vi "get shared memory structs and definitions.vi"(7 "engine in":refnum<class "Engine Parent Editor Node.lvclass">, 8 "error in (no error)":errorcluster, 11 "editor node in":refnum<class "module editor node.lvclass">) -> (0 "error out":errorcluster, 1 "shm file definitions":string, 2 "shm data structs":string, 3 "editor node out":refnum<class "module editor node.lvclass">, 5 "engine out":refnum<class "Engine Parent Editor Node.lvclass">)   [LabVIEW 2014, in "Shared Memory editor node.lvclass"]
uses:
  Shared Memory editor node.lvclass
  <vilib>/NI/DCAF/Tag Editor Core/Configuration Editor/Classes/Engine Parent/Engine Parent Editor Node.lvclass
  <vilib>/NI/DCAF/Tag Editor Core/Configuration Editor/Classes/Module editor node/module editor node.lvclass
  cheddar/C Header Generator.lvlib
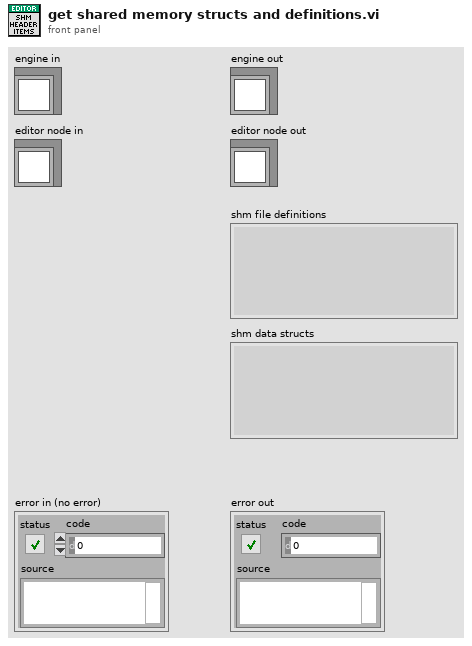
[diagram p1: front panel]
types:
  T1 = typedef "Shared Memory configuration.lvclass/Memory Allocation.ctl" = cluster{"shared memory name":string, "Lines":T2[]}
  T2 = typedef "Shared Memory configuration.lvclass/Line.ctl" = cluster{"channel":refnum<class "TBM channel.lvclass">}
  T3 = typedef "Shared Memory editor node.lvclass/define numeric params.ctl" = cluster{"name":string, "arg":i64}
  T4 = typedef "Shared Memory editor node.lvclass/struct params (single type).ctl" = cluster{"Struct name":string, "Data type":string, "Variable names":string[]}
  T5 = typedef "Shared Memory editor node.lvclass/define string params.ctl" = cluster{"name":string, "arg":string}
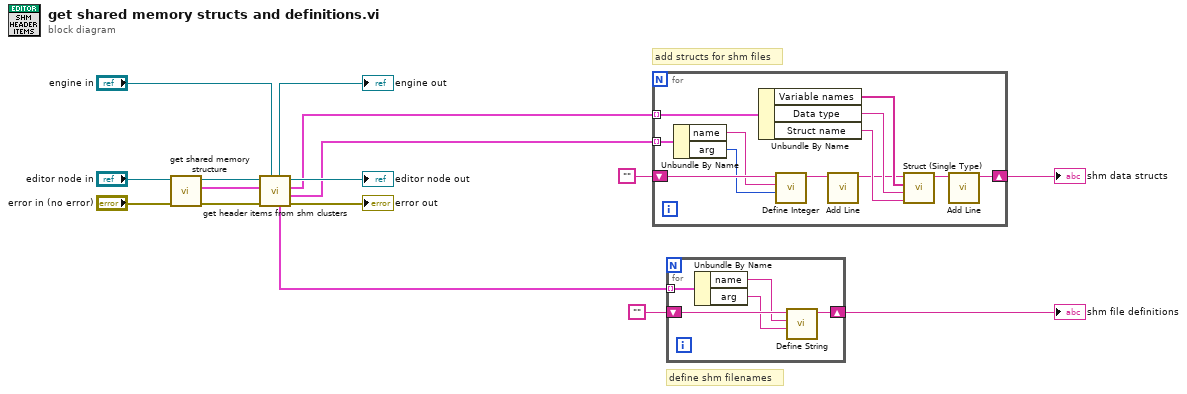
[diagram p0: block diagram]
diagram:
  # "add structs for shm files"
  # "define shm filenames"
  n1 = call "get shared memory structure.vi"("error in"="error in (no error)", "shared memory editor node"="editor node in") -> ("error out"=w14:errorcluster, "shm files"=w9:T1[], "shared memory editor node out"=w11:refnum<class "module editor node.lvclass">)  [unwired: 7 in]
  n2 = call "get header items from shm clusters.vi"("engine in"="engine in", "error in (no error)"=w14, "shm files"=w9, "module editor node in"=w11) -> ("error out"=→"error out":errorcluster, "numeric definitions"=w3:T3[], "structs"=w5:T4[], "module editor node out"=→"editor node out":refnum<class "module editor node.lvclass">, "string definitions"=w7:T5[], "engine out"=→"engine out":refnum<class "Engine Parent Editor Node.lvclass">)  [unwired: 2 in]
  n3 = for {
    tunnel: w5 -> [w28] mode=indexing
    shift-right: [w23] -> w2
    shift-left: "" -> [w22]
    tunnel: w3 -> [w19] mode=indexing
    n4 = Unbundle By Name(w19) -> ("name"=w17:string, "arg"=w18:i64)
    n5 = Unbundle By Name(w28) -> ("Variable names"=w27:string[], "Data type"=w26:string, "Struct name"=w25:string)
    n6 = call "Define Integer.vi"("Value"=w18, "Name"=w17, "String in"=w22) -> ("String out"=w21:string)  [unwired: 8 in]
    n7 = call "Add Line.vi"("String in"=w21) -> ("String out"=w20:string)  [unwired: 10 in]
    n8 = call "Struct (Single Type).vi"("Struct name"=w25, "Data type"=w26, "Variable names"=w27, "String in"=w20) -> ("String out"=w24:string)  [unwired: 7 in]
    n9 = call "Add Line.vi"("String in"=w24) -> ("String out"=w23:string)  [unwired: 10 in]
  }
  "shm data structs" <- w2
  n10 = for {
    tunnel: w7 -> [w33] mode=indexing
    shift-right: [w29] -> w1
    shift-left: "" -> [w32]
    n11 = Unbundle By Name(w33) -> ("name"=w30:string, "arg"=w31:string)
    n12 = call "Define String.vi"("Value"=w31, "Name"=w30, "String in"=w32) -> ("String out"=w29:string)  [unwired: 8 in]
  }
  "shm file definitions" <- w1
